vi "toScope3.vi"(8 "dt":dbl=0.1, 10 "error in":errorcluster, 11 "t0":dbl) -> (0 "error out":errorcluster, 3 "Shot #":string="1050")   [LabVIEW 2011]
uses:
  <vilib>/MDSplus/Library/MDSplus.lvlib
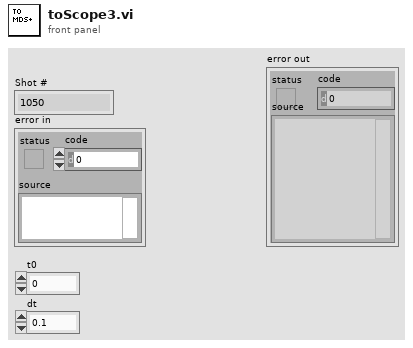
[diagram p1: front panel]
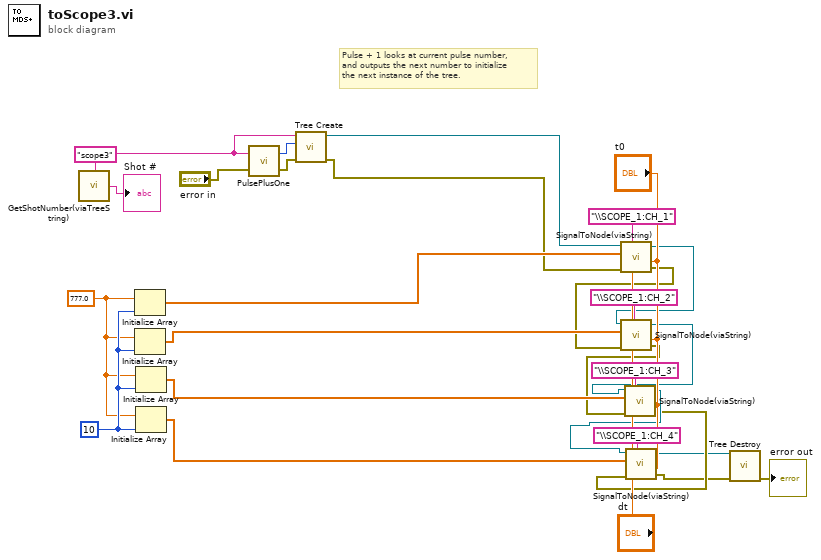
[diagram p0: block diagram]
diagram:
  w13 = "scope3"
  w27 = 777.0
  w28 = 10
  # "Pulse + 1 looks at current pulse number,\nand outputs the next number to initialize\nthe next instance of the tree."
  n1 = call "GetShotNumber(viaTreeString).vi"("Tree Name"=w13) -> ("Shot #"=→"Shot #":string)
  n2 = Initialize Array(w27, w28) -> (w26:dbl[])
  n3 = Initialize Array(w27, w28) -> (w25:dbl[])
  n4 = Initialize Array(w27, w28) -> (w24:dbl[])
  n5 = Initialize Array(w27, w28) -> (w23:dbl[])
  n6 = call "PulsePlusOne.vi"("error in"="error in", "Tree Name"=w13) -> ("error out"=w12:errorcluster, "Shot #"=w14:i32)
  n7 = call <vilib>:"Tree Create.vi"("error in (no error)"=w12, "Shot"=w14, "Name"=w13) -> ("error out"=w10:errorcluster, "Tree DVR out"=w11:refnum<data-value>)  [unwired: 7 in]
  n8 = call "SignalToNode(viaString).vi"("Tree DVR in"=w11, "NodePath"="\\SCOPE_1:CH_1", "y-axis (Data Range)"=w26, "Start Time"="t0", "Delta t"="dt", "error in (no error)"=w10) -> ("Tree DVR out"=w9:refnum<data-value>, "error out"=w8:errorcluster)  [unwired: 1 in]
  n9 = call "SignalToNode(viaString).vi"("Tree DVR in"=w9, "NodePath"="\\SCOPE_1:CH_2", "y-axis (Data Range)"=w25, "Start Time"="t0", "Delta t"="dt", "error in (no error)"=w8) -> ("Tree DVR out"=w7:refnum<data-value>, "error out"=w4:errorcluster)  [unwired: 1 in]
  n10 = call "SignalToNode(viaString).vi"("Tree DVR in"=w7, "NodePath"="\\SCOPE_1:CH_3", "y-axis (Data Range)"=w24, "Start Time"="t0", "Delta t"="dt", "error in (no error)"=w4) -> ("Tree DVR out"=w6:refnum<data-value>, "error out"=w5:errorcluster)  [unwired: 1 in]
  n11 = call "SignalToNode(viaString).vi"("Tree DVR in"=w6, "NodePath"="\\SCOPE_1:CH_4", "y-axis (Data Range)"=w23, "Start Time"="t0", "Delta t"="dt", "error in (no error)"=w5) -> ("Tree DVR out"=w3:refnum<data-value>, "error out"=w2:errorcluster)  [unwired: 1 in]
  n12 = call <vilib>:"Tree Destroy.vi"("error in (no error)"=w2, "Tree DVR in"=w3) -> ("error out"=→"error out":errorcluster)  [unwired: 9 in]
